vi "V-Cam Test.vi"() -> ()   [LabVIEW 2018]
uses:
  Hardware/Virtual Camera/Virtual Camera.lvclass
  C:/Program Files/National Instruments/LabVIEW 2018/vi.lib/ActorFramework/Actor/Actor.lvclass
  Type Defs/Virtual Camera Configuration.ctl
  Type Defs/Camera Type.ctl
  Type Defs/Physical Camera Assignment.ctl
  Type Defs/Camera Settings.ctl
  Hardware/Virtual Camera Messages/Virtual Camera Start Live Mode Msg/Virtual Camera Start Live Mode Msg.lvclass/Virtual Camera Start Live Mode Msg.ctl
  <vilib>/ActorFramework/Message Enqueuer/Message Enqueuer.lvclass/Message Enqueuer.ctl
  <vilib>/ActorFramework/Message Enqueuer/Enqueue.vi
  Hardware/Virtual Camera Messages/Virtual Camera Start Live Mode Msg/Virtual Camera Start Live Mode Msg.lvclass
  C:/Program Files/National Instruments/LabVIEW 2018/vi.lib/ActorFramework/Message/Message.lvclass
  Hardware/Virtual Camera Messages/Virtual Camera Stop Live Mode Msg/Virtual Camera Stop Live Mode Msg.lvclass
  <vilib>/ActorFramework/Stop Msg/Stop Msg.lvclass
  <vilib>/ActorFramework/Message Priority Queue/Priority Enqueue.vi
  GLOBAL/GLOBAL Time-critical.vi
  <vilib>/ActorFramework/Actor/Actor.lvclass
panel:
  out "Status":string
  in  "Camera Number":i32
  in  "Boolean":bool
  out "Intensity Graph":u16[][](graph)
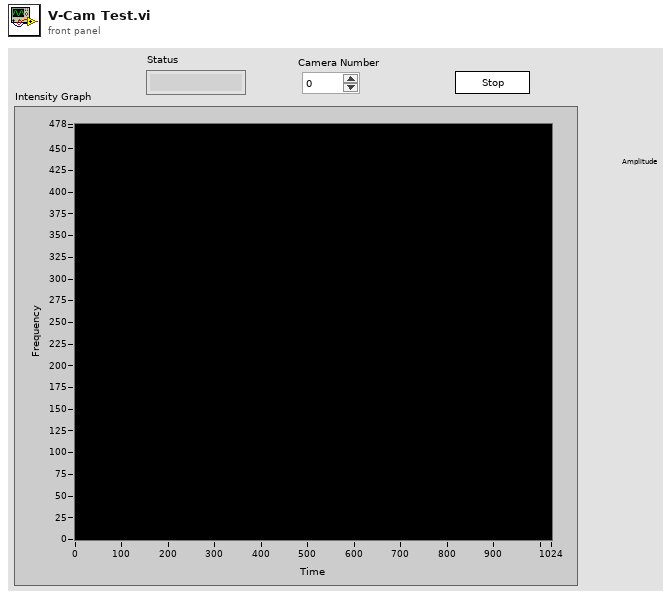
[diagram p1: front panel]
types:
  T1 = typedef "Camera Settings.ctl" = cluster{"Exposure Time (ms)":dbl, "Binning":enum16{"1x1", "2x2", "4x4"}, "Scan Mode (Flash)":enum16{"Fast", "Slow"}, "Trigger Mode (Flash)":enum16{"Fast", "Standard"}, "Frames to Acquire":dbl, "Pixel Correction (Flash)":bool}
  T2 = typedef "Virtual Camera Configuration.ctl" = cluster{"Camera Type":T3, "Active Cameras":T4[], "Sync Line":tag}
  T3 = typedef "Camera Type.ctl" = enum16{"Orca-Flash 4.0 V2"}
  T4 = typedef "Physical Camera Assignment.ctl" = cluster{"Channel Name":string, "Camera Type":T3, "Serial Number":string, "Flip Vertically":bool, "Flip Horizontally":bool}
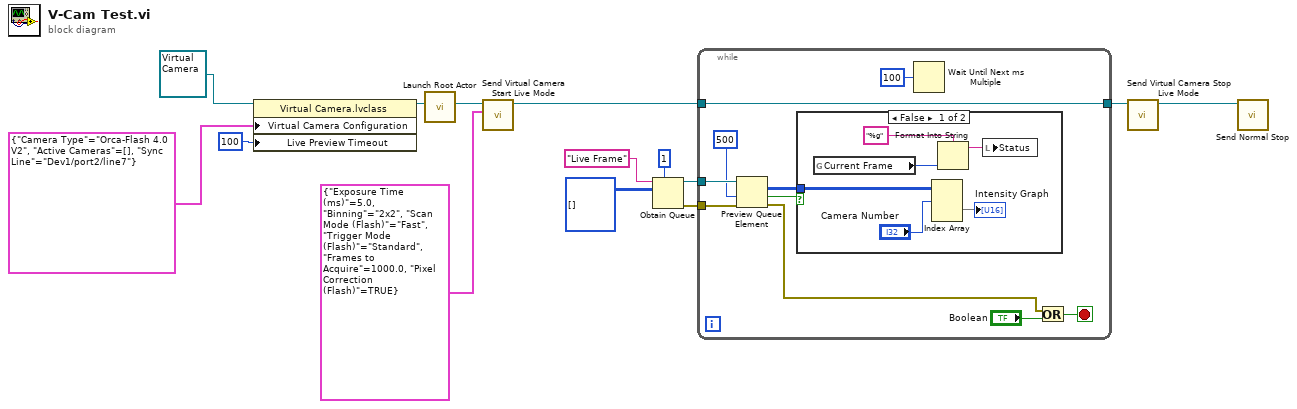
[diagram p0: block diagram]
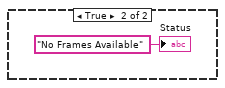
[diagram p2: hidden frame]
diagram:
  n1 = property class="Virtual Camera.lvclass"(reference=refnum<class "Virtual Camera.lvclass"> refnum ("Virtual Camera.lvlib:Virtual Camera.lvclass"), "Virtual Camera Configuration"=T2 {"Camera Type"=enum."Orca-Flash 4.0 V2", "Active Cameras"=[], "Sync Line"="Dev1/port2/line7"}, "Live Preview Timeout"=100) -> (reference out=w12:refnum<class "Virtual Camera.lvclass">)  [unwired: 1 in, 1 out]
  n2 = call <vilib>:"Launch Root Actor.vi"("Actor"=w12) -> ("Actor's Enqueuer"=w11:refnum<class "Message Enqueuer.lvclass">)  [unwired: 9 in, 1 out]
  n3 = call "Send Virtual Camera Start Live Mode.vi"("Camera Settings"=T1 {"Exposure Time (ms)"=5.0, "Binning"=enum."2x2", "Scan Mode (Flash)"=enum."Fast", "Trigger Mode (Flash)"=enum."Standard", "Frames to Acquire"=1000.0, "Pixel Correction (Flash)"=TRUE}, "Message Enqueuer"=w11) -> ("Message Enqueuer out"=w10:refnum<class "Message Enqueuer.lvclass">)  [unwired: 8 in, 1 out]
  n4 = Obtain Queue(max queue size (-1, unlimited)=1, name (unnamed)="Live Frame", element data type=u16[][][] [] ("element")) -> (queue out=w2:refnum<queue>, error out=w1:errorcluster)  [unwired: 2 in, 1 out]
  n5 = while {
    tunnel: w10 -> [w24]
    tunnel: [w24] -> w9
    tunnel: w2 -> [w22]
    tunnel: w1 -> [w21]
    stop <- w16 stop-if-true
    n6 = Preview Queue Element(queue=w22, timeout in ms (-1)=500, error in (no error)=w21) -> (element=w20:u16[][][], timed out?=w19:bool, error out=w15:errorcluster)  [unwired: 1 out]
    n7 = case shown="False" w19 {
      tunnel: w20 -> [w30 _]
      frame False {
        n8 = global read "GLOBAL Time-critical.vi" "Current Frame"() -> (w26:i32)
        n9 = Index Array(array=w30, index (dim 0)="Camera Number") -> (element=→"Intensity Graph":u16[][])  [unwired: 2 in]
        n10 = Format Into String(format string="%g", w26) -> (resulting string=w27:string)  [unwired: 2 in, 1 out]
        n11 = local write "Status"(w27) -> ()
      }
      frame True {
        "Status" <- "No Frames Available" ("Status")
      }
    }
    n12 = Wait Until Next ms Multiple(millisecond multiple=u32 100) -> ()  [unwired: 1 out]
    n13 = Or(x=w15, y="Boolean") -> (x .or. y?=w16:bool)
  }
  n14 = call "Send Virtual Camera Stop Live Mode.vi"("Message Enqueuer"=w9) -> ("Message Enqueuer out"=w8:refnum<class "Message Enqueuer.lvclass">)  [unwired: 9 in, 1 out]
  n15 = call <vilib>:"Send Normal Stop.vi"("Message Enqueuer"=w8) -> ()  [unwired: 10 in, 1 out]
